vi "flipY.vi"(11 "Array in":cluster{"a":dbl, dbl}[](array[cluster])) -> (3 "Array out":cluster{"a":dbl, dbl}[](array[cluster]))   [LabVIEW 2020]
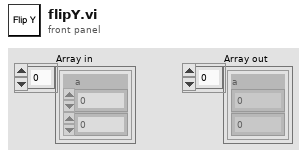
[diagram p1: front panel]
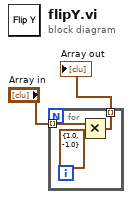
[diagram p0: block diagram]
diagram:
  n1 = for {
    tunnel: "Array in" -> [w5] mode=indexing
    tunnel: [w3] -> w2 mode=indexing
    n2 = Multiply(x=w5, y=cluster{"a":dbl, dbl} {"a"=1.0, -1.0}) -> (x*y=w3:cluster{"a":dbl, dbl})
  }
  "Array out" <- w2
